vi "Time series data viewer larger window menu.vi"(8 "error in (no error)":errorcluster, 11 "menu":refnum<k9>) -> (0 "error out":errorcluster, 3 "menu reference out":refnum<k9>)   [LabVIEW 2020]
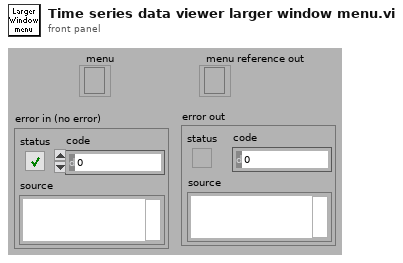
[diagram p1: front panel]
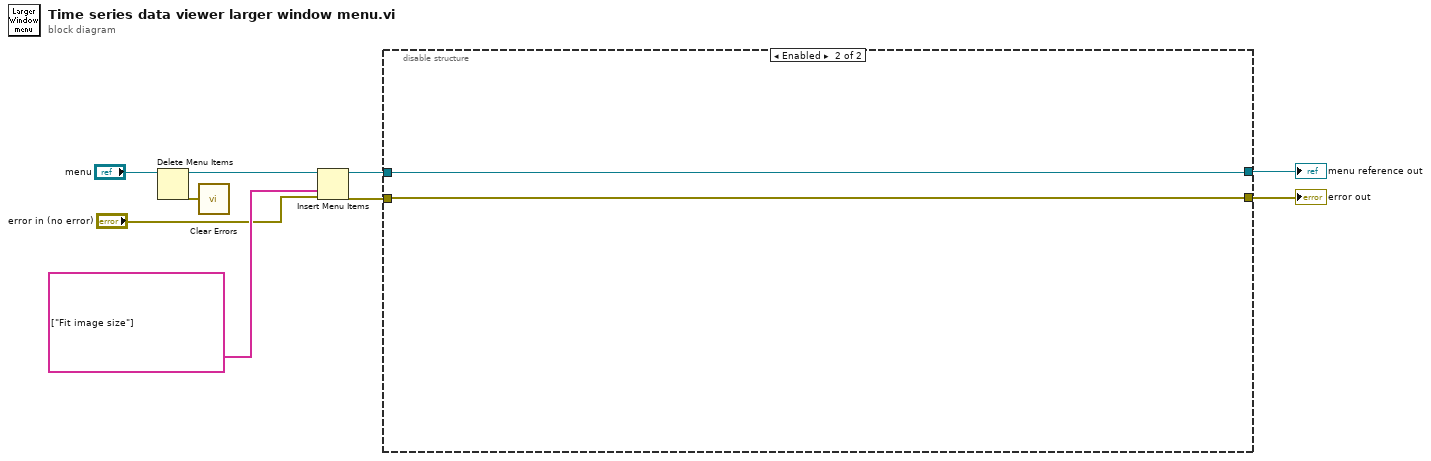
[diagram p0: block diagram]
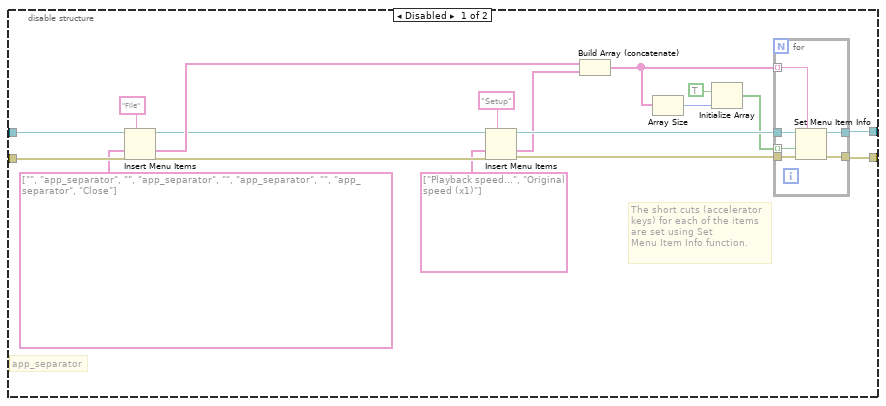
[diagram p2: hidden frame]
diagram:
  n1 = Delete Menu Items(9:"menu") -> (0:w3:errorcluster, 3:w6:refnum<k9>)  [unwired: 2 in, 1 out]
  n2 = call <vilib>:"Clear Errors.vi"("error in (no error)"=w3) -> ()  [unwired: 5 in, 2 out]
  n3 = Insert Menu Items(6:"error in (no error)", 7:string[] ["Fit image size"] ("item tags"), 9:w6) -> (0:w8:errorcluster, 3:w4:refnum<k9>)  [unwired: 4 out]
  n4 = disable-structure shown="Enabled" {
    disable-tunnel: [w27 w34] -> w9
    disable-tunnel: w8 -> [w25 w34]
    disable-tunnel: [w22 w35] -> w5
    disable-tunnel: w4 -> [w19 w35]
    frame Disabled {
      # "The short cuts (accelerator\nkeys) for each of the items\nare set using Set\nMenu Item Info function."
      # "app_separator"
      n5 = Insert Menu Items(5:"File" ("menu tag"), 6:w25, 7:string[] ["", "app_separator", "", "app_separator", "", "app_separator", "", "app_separator", "Close"] ("item tags"), 9:w19) -> (0:w26:errorcluster, 1:w24:string[], 3:w20:refnum<k9>)  [unwired: 2 out]
      n6 = Insert Menu Items(5:"Setup" ("menu tag"), 6:w26, 7:string[] ["Playback speed...", "Original speed (x1)"] ("item tags"), 9:w20) -> (0:w18:errorcluster, 1:w16:string[], 3:w17:refnum<k9>)  [unwired: 2 out]
      n7 = Build Array (concatenate)(w24, w16) -> (w13:string[])
      n8 = Array Size(array=w13) -> (size(s)=w15:i32)
      n9 = Initialize Array(TRUE, w15) -> (w14:bool[])
      n10 = for {
        tunnel: w17 -> [w33]
        tunnel: [w32] -> w22
        tunnel: w13 -> [w31] mode=indexing
        tunnel: w18 -> [w30]
        tunnel: [w29] -> w27
        tunnel: w14 -> [w28] mode=indexing
        n11 = Set Menu Item Info(7:w31, 8:w30, 9:w28, 11:w33) -> (0:w29:errorcluster, 3:w32:refnum<k9>)  [unwired: 1 in, 2 out]
      }
    }
    frame Enabled {
    }
  }
  "error out" <- w9
  "menu reference out" <- w5
